vi "QWinJumpListItem.vi"(8 "Error In":errorcluster, 10 "type":T1 items=["Destination", "Link", "Separator"]) -> (0 "Error Out":errorcluster, 3 "New QWinJumpListItem":refnum<class "QWinJumpListItem.lvclass">)   [LabVIEW 2014, in "QWinJumpListItem.lvclass"]
doc: "LabVIEW-specific documentation is not yet available."
uses:
  QWinJumpListItem.lvclass
  Type.ctl
  LQ Core/LQCoreEngine/_Internal/LQIdentity Registry Action.ctl
  LQ Core/LQIdentity/LQIdentity.lvclass/LQIdentity.ctl
  LQ Core/LQCoreEngine/LQCoreEngine.lvclass
  LQ Core/LQ Core.lvlib
  LQ Core/LQIdentity/LQIdentity.lvclass
panel:
  # "Copyright (c) 2016 Sze Howe Koh\n\nThis Source Code Form is subject to the terms of the Mozilla Public\nLicense, v. 2.0. If a copy of the MPL was not distributed with this\nfile, You can obtain one at http://mozilla.org/MPL/2.0/."
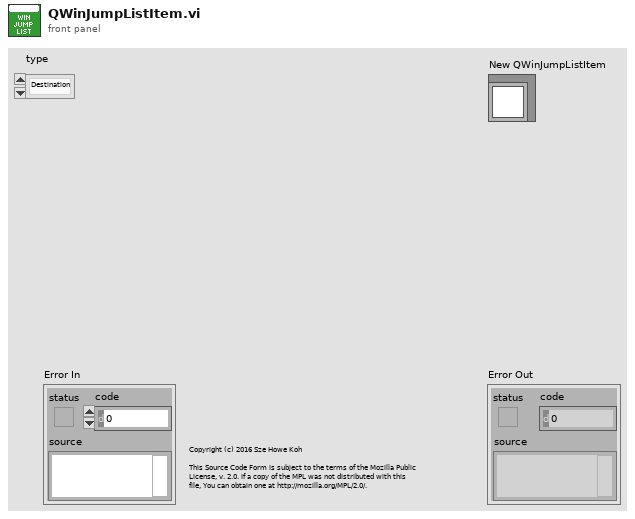
[diagram p1: front panel]
types:
  T1 = typedef "QWinJumpListItem.lvclass/Type.ctl" = i32
  T2 = typedef "LQ Core.lvlib/LQCoreEngine.lvclass/LQIdentity Registry Action.ctl" = enum16{"Init", "Register LQIdentity", "Get LQIdentity Info", "Deregister LQIdentity"}
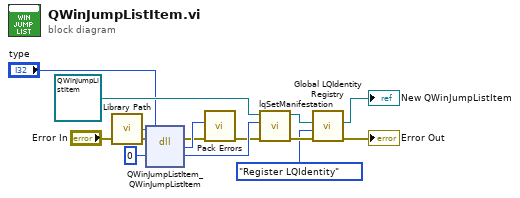
[diagram p0: block diagram]
diagram:
  n1 = call "Library Path.vi"() -> ("Library Path"=w11:path)
  n2 = dll-call lib="?" fn="QWinJumpListItem_QWinJumpListItem"(path in=w11, error in="Error In", "_retVal"=u64 0 ("_instance"), "type"="type") -> (error out=w9:errorcluster, w10:i32, "_retVal"=w12:u64)  [unwired: 2 in, 1 out]
  n3 = call "Pack Errors.vi"("Error In"=w9, "Error Code"=w10) -> ("Error Out"=w8:errorcluster)  [unwired: 9 in]
  n4 = call "lqSetManifestation.vi"("Error In"=w8, "Manifestation"=w12, "LQIdentity in"=refnum<class "QWinJumpListItem.lvclass"> refnum ("QWinJumpListItem")) -> ("Error Out"=w6:errorcluster, "LQIdentity out"=w7:refnum<class "QWinJumpListItem.lvclass">)  [unwired: 7 in]
  n5 = call "Global LQIdentity Registry.vi"("Error In"=w6, "Registry Action"=LQIdentity_Registry_Action."Register LQIdentity", "LQIdentity Info In"=w7) -> ("Error Out"=→"Error Out":errorcluster, "LQIdentity Info Out"=→"New QWinJumpListItem":refnum<class "QWinJumpListItem.lvclass">)  [unwired: 7 in]
